vi "CTRE_Phoenix_CANdle_FireAnimation.vi"(0 "CTRE_CANdle_DeviceRef":T1, 1 "Sparking":dbl=1.0 min=0.0 max=1.0 step=0.0001, 2 "Cooling":dbl=1.0 min=0.0 max=1.0 step=0.0001, 5 "Speed":dbl=1.0 min=0.0 max=1.0 step=0.0001, 7 "Num LED":i32=-1, 9 "Brightness":dbl=1.0 min=0.0 max=1.0 step=0.0001, 11 "error in":errorcluster) -> (4 "CTRE_CANdle_DeviceRef":T1, 15 "error out":errorcluster)   [LabVIEW 2020]
doc: "Animation that looks similar to a flame flickering\n\n<b>Speed</b> adjust the speed [0,1] at which the animation runs. Valid values range from 0 to 1 where 1 is the fastest animation speed.\n\n<b>Num LEDs</b> defines the total number of LEDs to use for the animation.\n\n<b>Brightness</b> defintes how bright the animation will be [0,1]\n\n<b>Sparking</b> is the rate at which the animated fire \"sparks\" [0,1]\n\n<b>Cooling</b> is the rate at which the animated fire \"cools\" along the travel [0,1]"
uses:
  <vilib>/Rock Robotics/WPI/ThirdParty/Phoenix-LabVIEW/CANdle/Controls/CTRE_Phoenix_CANdle_DeviceRef.ctl
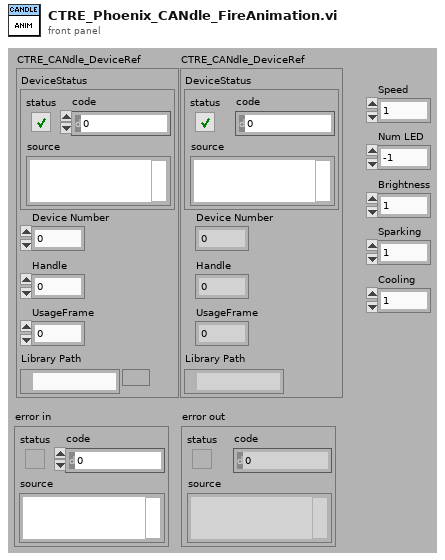
[diagram p1: front panel]
types:
  T1 = typedef "CTRE_Phoenix_CANdle_DeviceRef.ctl" = cluster{"DeviceStatus":errorcluster, "Device Number":u8, "Handle":u64, "UsageFrame":u32, "Library Path":path}
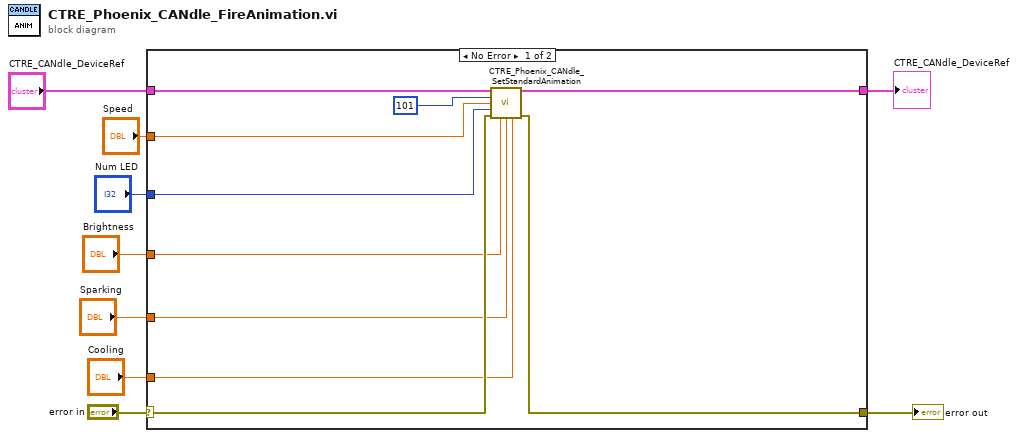
[diagram p0: block diagram]
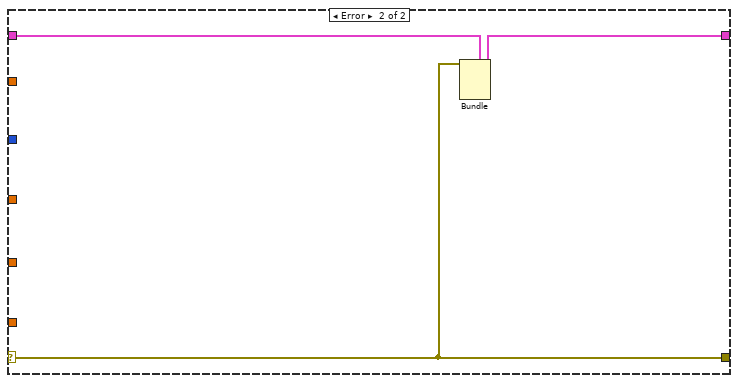
[diagram p2: hidden frame]
diagram:
  n1 = case shown="No Error" "error in" {
    selector: "error in" -> [w15 w21]
    tunnel: "CTRE_CANdle_DeviceRef" -> [w19 w22]
    tunnel: [w14 w21] -> w9
    tunnel: [w13 w20] -> w6
    tunnel: "Speed" -> [w17 _]
    tunnel: "Num LED" -> [w16 _]
    tunnel: "Brightness" -> [w12 _]
    tunnel: "Sparking" -> [w11 _]
    tunnel: "Cooling" -> [w10 _]
    frame No Error {
      n2 = call <vilib>:"CTRE_Phoenix_CANdle_SetStandardAnimation.vi"("CTRE_CANdle_DeviceRef"=w19, "idx"=101, "speed"=w17, "numLED"=w16, "error in"=w15, "brightness"=w12, "param4"=w11, "param5"=w10) -> ("CTRE_CANdle_DeviceRef"=w13:T1, "error out"=w14:errorcluster)  [unwired: 6 in]
    }
    frame Error {
      n3 = Bundle(cluster=w22, "DeviceStatus"=w21) -> (w20:T1)  [unwired: 4 in]
    }
  }
  "error out" <- w9
  "CTRE_CANdle_DeviceRef" <- w6
